vi "kloehn V6 - Write - Read.vi"(10 "Send String":string, 11 "kloehn session in":T1={"VISA resource out"="COM12", "error out"={"status"=FALSE, "code"=0, "source"=""}}) -> (1 "Unparsed Response String":string, 2 "Parsed Response String":string, 3 "kloehn session out":T1={"VISA resource out"="COM12", "error out"={"status"=FALSE, "code"=0, "source"=""}}, 5 "Status":enum16{"Ready", "Busy"}(ring))   [LabVIEW 2010]
doc: "From user Slipknot on LV forums"
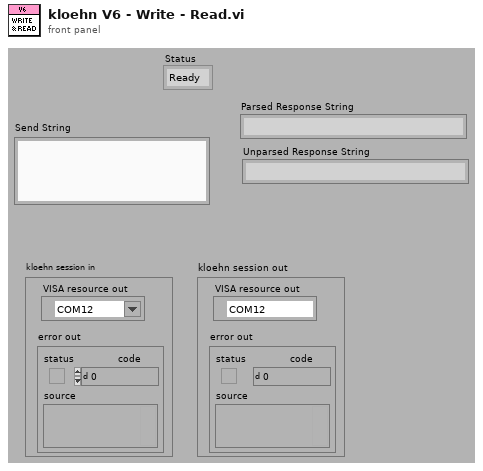
[diagram p1: front panel]
types:
  T1 = cluster{"VISA resource out":refnum<visa-resource-name>, "error out":errorcluster}
  T2 = cluster{"VISA resource out":refnum<visa-resource-name>, "error IO":errorcluster}
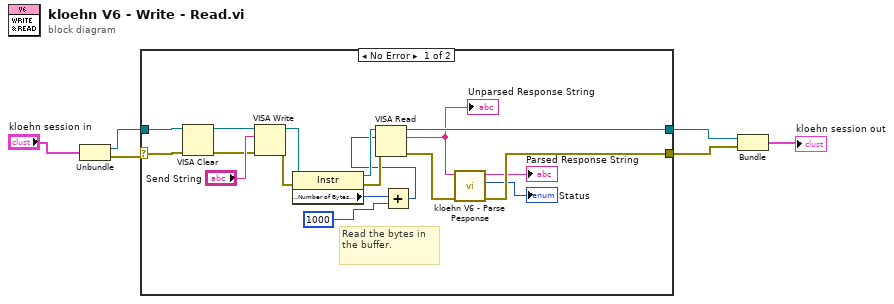
[diagram p0: block diagram]
diagram:
  n1 = Unbundle("kloehn session in") -> ("VISA resource out"=w5:refnum<visa-resource-name>, "error out"=w4:errorcluster)
  n2 = case shown="No Error" w4 {
    selector: w4 -> [w23 w26]
    tunnel: w5 -> [w22 w25]
    tunnel: [w16 w26] -> w2
    tunnel: [w19 w25] -> w3
    frame No Error {
      # "Read the bytes in the buffer."
      n3 = VISA Clear(VISA resource name=w22, error in (no error)=w23) -> (VISA resource name out=w20:refnum<visa-resource-name>, error out=w21:errorcluster)
      n4 = VISA Write(VISA resource name=w20, write buffer="Send String", error in (no error)=w21) -> (VISA resource name out=w11:refnum<visa-resource-name>, error out=w9:errorcluster)  [unwired: 1 out]
      n5 = property class="Instr"(reference=w11, error in=w9) -> (reference out=w10:refnum<visa-resource-name>, error out=w8:errorcluster, "Serial Settings:Number of Bytes at Serial Port"=w13:u32)
      n6 = Add(x=w13, y=1000) -> (x+y=w7:u32)
      n7 = VISA Read(VISA resource name=w10, byte count=w7, error in (no error)=w8) -> (VISA resource name out=w19:refnum<visa-resource-name>, read buffer=w18:string, error out=w17:errorcluster)  [unwired: 1 out]
      "Unparsed Response String" <- w18
      n8 = call "kloehn V6 - Parse Pesponse.vi"("error in"=w17, "Response String"=w18) -> ("error out"=w16:errorcluster, "Status"=→"Status":enum16{"Ready", "Busy"}, "Response String"=→"Parsed Response String":string)  [unwired: 7 in]
    }
    frame Error {
    }
  }
  n9 = Bundle("VISA resource out"=w3, "error IO"=w2) -> (→"kloehn session out":T2)  [unwired: 1 in]
